vi "Assign Value.vi"(8 "error in (no error)":errorcluster, 10 "Assigned Value":refnum<class "Abs_Value.lvclass">, 11 "Abs_String in":refnum<class "Abs_String 1D.lvclass">) -> (0 "error out":errorcluster, 3 "Abs_String out":refnum<class "Abs_String 1D.lvclass">)   [LabVIEW 2021, in "Abs_String 1D.lvclass"]
uses:
  Abs_String 1D.lvclass
  Value/Abs_Value.lvclass
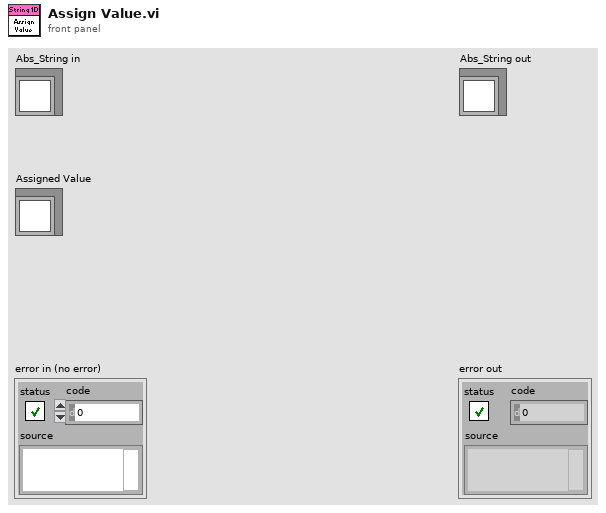
[diagram p1: front panel]
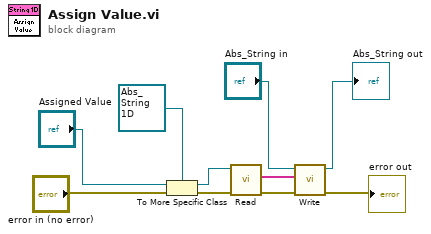
[diagram p0: block diagram]
diagram:
  n1 = To More Specific Class(target class=refnum<class "Abs_String 1D.lvclass"> refnum ("Abs_String.lvclass"), reference="Assigned Value", error in="error in (no error)") -> (specific class reference=w6:refnum<class "Abs_String 1D.lvclass">, error out=w7:errorcluster)
  n2 = call-dynamic "Read.vi"("error in (no error)"=w7, "Abs_String in"=w6) -> ("error out"=w5:errorcluster, "Array"=w4:string[])  [unwired: 7 in, 1 out]
  n3 = call-dynamic "Write.vi"("error in (no error)"=w5, "Array"=w4, "Abs_String in"="Abs_String in") -> ("error out"=→"error out":errorcluster, "Abs_String out"=→"Abs_String out":refnum<class "Abs_String 1D.lvclass">)  [unwired: 7 in]
